vi "count_integrations.vi"(3 "error in":errorcluster, 5 "Plan":string) -> (0 "error out":errorcluster, 2 "integrals required":i32)   [LabVIEW 2020]
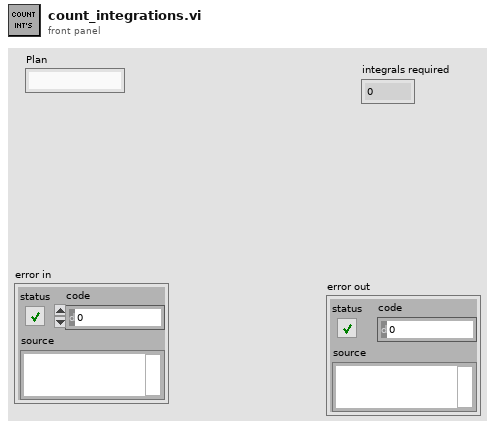
[diagram p1: front panel]
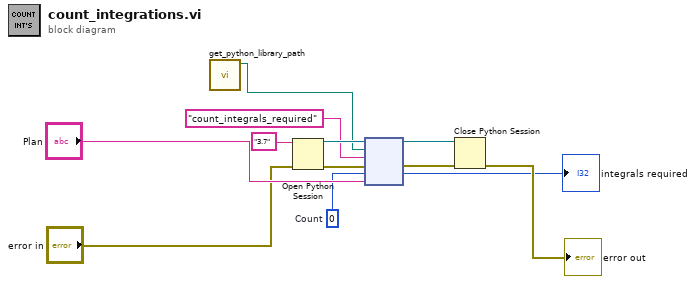
[diagram p0: block diagram]
diagram:
  w3 = 0  # Count
  n1 = call "get_python_library_path.vi"() -> ("Python library path"=w1:path)  [unwired: 11 in]
  n2 = Open Python Session(python version="3.7" ("Python version"), 3:"error in") -> (session out=w11:refnum<k35>, error out=w9:errorcluster)  [unwired: 1 in]
  n3 = node(w11, w1, "count_integrals_required" ("function name"), w9, w3, "Plan") -> (w7:refnum<k35>, w6:errorcluster, →"integrals required":i32)  [unwired: 1 in, 2 out]
  n4 = Close Python Session(session in=w7, error in=w6) -> (11:→"error out":errorcluster)
